vi "Find Max Hypotenuse or 1.vi"(1 "constants":cluster{"a":dbl, "b":dbl, "c":dbl, "d":dbl}) -> (0 "Max or 1":dbl)   [LabVIEW 2016, in "Huskie Swerve.lvlib"]
uses:
  Huskie Swerve.lvlib
  <vilib>/ptbypt/NI_PtbyPt.lvlib
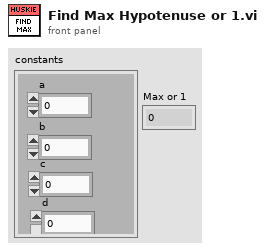
[diagram p1: front panel]
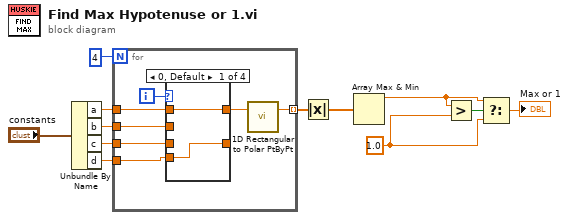
[diagram p0: block diagram]
diagram:
  w5 = 1.0 ("y")
  n1 = Unbundle By Name("constants") -> ("a"=w10:dbl, "b"=w9:dbl, "c"=w8:dbl, "d"=w7:dbl)
  n2 = for {
    N: 4 -> [_]
    tunnel: w10 -> [w18]
    tunnel: w9 -> [w16]
    tunnel: w8 -> [w15]
    tunnel: w7 -> [w14]
    tunnel: [w13] -> w2 mode=indexing
    i -> [w19]
    n3 = case shown="0, Default" w19 {
      tunnel: [w21 w23 w25 w26] -> w17
      tunnel: w18 -> [w21 w23 _ _]
      tunnel: w16 -> [_ _ w25 w26]
      tunnel: w15 -> [_ w22 w24 _]
      tunnel: [w20 w22 w24 w27] -> _
      tunnel: w14 -> [w20 _ _ w27]
      frame 0, Default {
      }
      frame 1 {
      }
      frame 2 {
      }
      frame 3 {
      }
    }
    n4 = call <vilib>:"1D Rectangular to Polar PtByPt.vi"("x"=w17) -> ("magnitude"=w13:dbl)  [unwired: 1 in, 1 out]
  }
  n5 = Absolute Value(x=w2) -> (abs(x)=w1:dbl[])
  n6 = Array Max & Min(array=w1) -> (max value=w3:dbl)  [unwired: 3 out]
  n7 = Greater?(x=w3, y=w5) -> (0:w6:bool)
  n8 = Select(t=w3, s=w6, f=w5) -> (s? t:f=→"Max or 1":dbl)
